vi "Expression Format Example.vi"() -> ()   [LabVIEW 2020, in "Logger Examples.lvlib"]
uses:
  <vilib>/gpm_packages/@cs/event-logger/Examples/Logger Examples.lvlib
  <vilib>/gpm_packages/@cs/event-logger/Source/Composed Log/Types/Log Level.ctl
  <vilib>/gpm_packages/@cs/event-logger/Source/String Formats/String Expression Format/String Expression Format.lvclass/String Expression Format.ctl
  <vilib>/gpm_packages/@cs/event-logger/Source/Composed Log/LoggerReference/LoggerReference.lvclass/LoggerReference.ctl
  601d143e-8928-4a3b-9174-3083e729aaa9.vi
  <vilib>/gpm_packages/@cs/event-logger/Source/String Formats/String Expression Format/Run Formatter.vi
  <vilib>/gpm_packages/@cs/event-logger/Source/Composed Log/LoggerReference/Return Aggregate Queues.vi
  <vilib>/gpm_packages/@cs/event-logger/Source/Composed Log/LoggerReference/Add Aggregate Log.vi
  601d143e-8928-4a3b-9174-3083e729aaa9.vi/f15837f3-2100-4c7f-976a-c76a45bfaa57.vi
  <vilib>/gpm_packages/@cs/event-logger/Source/Composed Log/LoggerReference/Log.vi
  <vilib>/gpm_packages/@cs/event-logger/Source/Composed Log/LoggerReference/Get Valid Event Time.vi
  <vilib>/dlg_ctls.llb/Space Constant.vi
  <vilib>/gpm_packages/@cs/event-logger/Source/Composed Log/LoggerReference/Send Add Sink.vi
  <vilib>/gpm_packages/@cs/event-logger/Source/Composed Log/LoggerReference/Remove Stale Logs.vi
  <vilib>/gpm_packages/@cs/event-logger/Source/String Formats/String Expression Format/String Expression Format.lvclass
  C:/Program Files/National Instruments/LabVIEW 2020/vi.lib/gpm_packages/@cs/event-logger/Source/IStringFormat/IStringFormat.lvclass
  <vilib>/gpm_packages/@cs/event-logger/Source/Text File Sink/Text File Sink.lvclass
  C:/Program Files/National Instruments/LabVIEW 2020/vi.lib/gpm_packages/@cs/event-logger/Source/String Log Sink/String Log Sink.lvclass
  <vilib>/gpm_packages/@cs/event-logger/Source/String Control Sink/String Control Sink.lvclass
  <vilib>/gpm_packages/@cs/event-logger/Source/String Log Sink/String Log Sink.lvclass
  C:/Program Files/National Instruments/LabVIEW 2020/vi.lib/gpm_packages/@cs/event-logger/Source/Composed Log/Log Sink/Log Sink.lvclass
  <vilib>/gpm_packages/@cs/event-logger/Source/Composed Log/Application Logger/Launch Worker Loop.vi
  <vilib>/gpm_packages/@cs/event-logger/Source/Composed Log/LoggerReference/Initialize Logger Instance.vi
  <vilib>/gpm_packages/@cs/event-logger/Source/Composed Log/LoggerReference/LoggerReference.lvclass
  <vilib>/gpm_packages/@cs/event-logger/Source/Composed Log/IErrorFormat/IErrorFormat.lvclass
  <vilib>/gpm_packages/@cs/event-logger/Source/Composed Log/Log Sink/Log Sink.lvclass
  <vilib>/gpm_packages/@cs/event-logger/Source/Composed Log/Composed Log.lvlib
  <vilib>/gpm_packages/@cs/event-logger/Source/Composed Log/ILogFilter/ILogFilter.lvclass
panel:
  in  "Log Error":bool
  in  "Error Information":string
  in  "Error Code":i32
  in  "Event Level":T1(ring)
  out "Event - %s[EVT]  - Occured at <%T>[TIME] From %s[ID], Level %s[LVL]":string
  out "%<%A at %H:%M:%S>T[TIME] -- %s[EVT]":string
  out "<%T>[TIME]<%s[LVL]-%s[ID]><%s>[EVT]":string
  in  "Data To Log":string
  in  "Source":string="User"
  in  "Log":bool
  # "Run the VI. Note the different formats - each string indicator is displaying the same event with different string format."
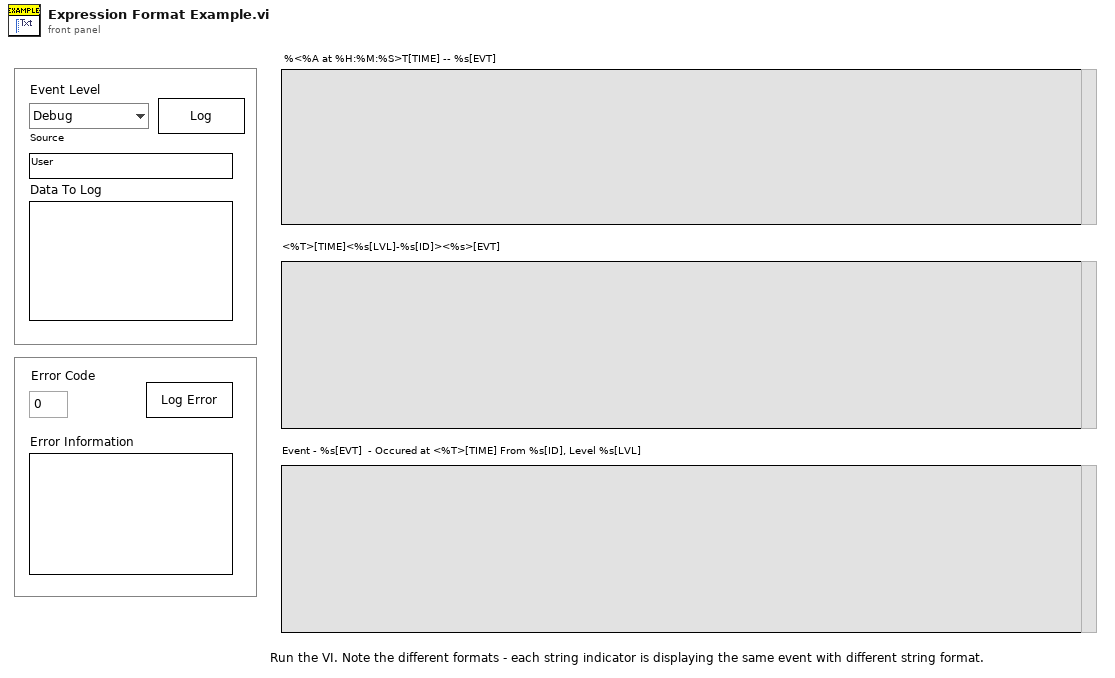
[diagram p1: front panel]
types:
  T1 = enum16{"Debug", "Info", "Warning", "Error", "Critical"}
  T2 = typedef "Composed Log.lvlib/Log Level.ctl" = enum16{"Debug", "Info", "Warning", "Error", "Critical"}
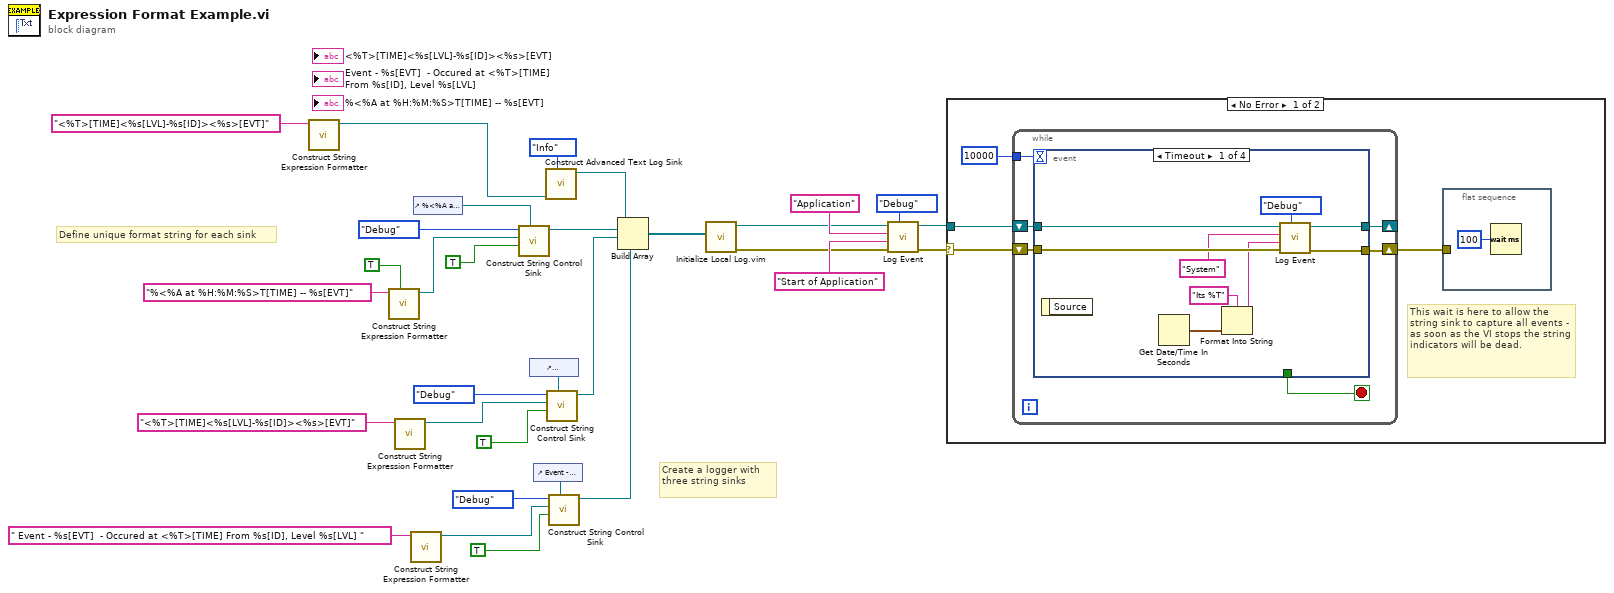
[diagram p0: block diagram]
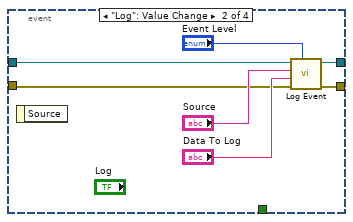
[diagram p2: hidden frame]
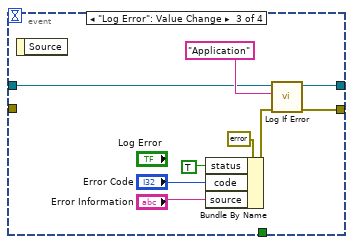
[diagram p3: hidden frame]
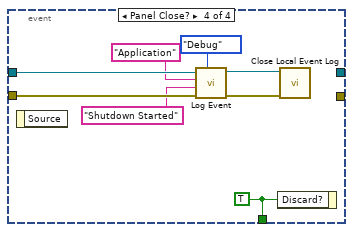
[diagram p4: hidden frame]
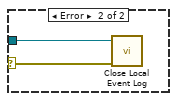
[diagram p5: hidden frame]
diagram:
  # "Define unique format string for each sink"
  # "Create a logger with three string sinks"
  n1 = call <vilib>:"Construct String Expression Formatter.vi"("Format Specifier"="<%T>[TIME]<%s[LVL]-%s[ID]><%s>[EVT]") -> ("String Expression Format out"=w1:refnum<class "String Expression Format.lvclass">)  [unwired: 9 in, 1 out]
  n2 = call <vilib>:"Construct String Expression Formatter.vi"("Append EOL?"=TRUE, "Format Specifier"="%<%A at %H:%M:%S>T[TIME] -- %s[EVT]") -> ("String Expression Format out"=w14:refnum<class "String Expression Format.lvclass">)  [unwired: 8 in, 1 out]
  n3 = call <vilib>:"Construct String Expression Formatter.vi"("Format Specifier"="<%T>[TIME]<%s[LVL]-%s[ID]><%s>[EVT]") -> ("String Expression Format out"=w11:refnum<class "String Expression Format.lvclass">)  [unwired: 9 in, 1 out]
  n4 = call <vilib>:"Construct String Expression Formatter.vi"("Format Specifier"=" Event - %s[EVT]  - Occured at <%T>[TIME] From %s[ID], Level %s[LVL] ") -> ("String Expression Format out"=w7:refnum<class "String Expression Format.lvclass">)  [unwired: 9 in, 1 out]
  n5 = control-ref of="%<%A at %H:%M:%S>T[TIME] -- %s[EVT]"() -> (w27:refnum<vi>)
  n6 = call <vilib>:"Construct String Control Sink.vi"("Str Refnum"=w27, "AutoScroll?(F)"=TRUE, "LogFormat"=w14, "LogLevel"=Log_Level."Debug") -> ("String Control Sink out"=w22:refnum<class "String Control Sink.lvclass">)  [unwired: 7 in]
  n7 = control-ref of="<%T>[TIME]<%s[LVL]-%s[ID]><%s>[EVT]"() -> (w29:refnum<vi>)
  n8 = control-ref of="Event - %s[EVT]  - Occured at <%T>[TIME] From %s[ID], Level %s[LVL]"() -> (w23:refnum<vi>)
  n9 = call <vilib>:"Construct Advanced Text Log Sink.vi"("LogLevel"=Log_Level."Info", "StringFormat"=w1) -> ("Text File Sink out"=w4:refnum<class "Text File Sink.lvclass">)  [unwired: 9 in]
  n10 = call <vilib>:"Construct String Control Sink.vi"("Str Refnum"=w29, "AutoScroll?(F)"=TRUE, "LogFormat"=w11, "LogLevel"=Log_Level."Debug") -> ("String Control Sink out"=w10:refnum<class "String Control Sink.lvclass">)  [unwired: 7 in]
  n11 = call <vilib>:"Construct String Control Sink.vi"("Str Refnum"=w23, "AutoScroll?(F)"=TRUE, "LogFormat"=w7, "LogLevel"=Log_Level."Debug") -> ("String Control Sink out"=w6:refnum<class "String Control Sink.lvclass">)  [unwired: 7 in]
  n12 = Build Array(w4, w22, w10, w6) -> (w5:refnum<class "String Log Sink.lvclass">[])
  n13 = call "Initialize Local Log.vim"("Startup Sink(s)"=w5) -> ("error out"=w18:errorcluster, "Log Instance Reference"=w17:refnum<class "LoggerReference.lvclass">)  [unwired: 8 in, 1 out]
  n14 = call <vilib>:"Log Event.vi"("Event Level"=Log_Level."Debug", "error in (no error)"=w18, "Data To Log"="Start of Application", "SourceID"="Application", "Log Instance"=w17) -> ("error out"=w16:errorcluster, "Log Instance Out"=w15:refnum<class "LoggerReference.lvclass">)  [unwired: 5 in]
  n15 = case shown="No Error" w16 {
    selector: w16 -> [w34 w76]
    tunnel: w15 -> [w35 w77]
    frame No Error {
      # "This wait is here to allow the string sink to capture all events - as soon as the VI stops the string indicators will be dead."
      n16 = while {
        shift-right: [w40] -> _
        shift-left: w35 -> [w41]
        shift-right: [w38] -> w32
        shift-left: w34 -> [w39]
        tunnel: 10000 -> [w37]
        stop <- w42 stop-if-true
        n17 = event shown="[0] Timeout" {
          selector: _ -> [_ _ _ _]
          dyn-events: _ -> [_ _ _ _]
          timeout: w37 -> [_ _ _ _]
          tunnel: [_ _ _ w75] -> w42
          tunnel: w41 -> [w51 w55 w61 w73]
          tunnel: [w50 w53 w59 _] -> w40
          tunnel: w39 -> [w48 w52 _ w74]
          tunnel: [w47 w54 w60 _] -> w38
          event Timeout {
            n18 = event-data() -> ()  [unwired: 1 in, 1 out]
            n19 = Get Date/Time In Seconds() -> (seconds since 1Jan1904=w45:timestamp)
            n20 = Format Into String(format string="Its %T" ("Log Message"), w45) -> (resulting string=w43:string)  [unwired: 2 in, 1 out]
            n21 = call <vilib>:"Log Event.vi"("Event Level"=Log_Level."Debug", "error in (no error)"=w48, "Data To Log"=w43, "SourceID"="System" ("Event Source"), "Log Instance"=w51) -> ("error out"=w47:errorcluster, "Log Instance Out"=w50:refnum<class "LoggerReference.lvclass">)  [unwired: 5 in]
          }
          event "Log": Value Change {
            n22 = event-data() -> ()  [unwired: 1 in, 1 out]
            n23 = call <vilib>:"Log Event.vi"("Event Level"="Event Level", "error in (no error)"=w52, "Data To Log"="Data To Log", "SourceID"="Source", "Log Instance"=w55) -> ("error out"=w54:errorcluster, "Log Instance Out"=w53:refnum<class "LoggerReference.lvclass">)  [unwired: 5 in]
          }
          event "Log Error": Value Change {
            n24 = event-data() -> ()  [unwired: 1 in, 1 out]
            n25 = Bundle By Name(cluster=errorcluster {"status"=FALSE, "code"=0, "source"=""} ("Error In"), "status"=TRUE, "code"="Error Code", "source"="Error Information") -> (w65:errorcluster)
            n26 = call <vilib>:"Log If Error.vi"("Error In"=w65, "SourceID"="Application" ("Source"), "Log Instance"=w61) -> ("error out"=w60:errorcluster, "Log Instance Out"=w59:refnum<class "LoggerReference.lvclass">)  [unwired: 7 in]
          }
          event Panel Close? {
            w75 = TRUE ("Discard?")
            n27 = event-data() -> ()  [unwired: 1 in, 1 out]
            n28 = call <vilib>:"Log Event.vi"("Event Level"=Log_Level."Debug", "error in (no error)"=w74, "Data To Log"="Shutdown Started", "SourceID"="Application", "Log Instance"=w73) -> ("error out"=w72:errorcluster, "Log Instance Out"=w71:refnum<class "LoggerReference.lvclass">)  [unwired: 5 in]
            n29 = event-data("Discard?"=w75) -> ()  [unwired: 1 in, 1 out]
            n30 = call <vilib>:"Close Local Event Log.vi"("error in (no error)"=w72, "Log Instance"=w71) -> ()  [unwired: 9 in, 1 out]
          }
        }
      }
      n31 = flat-sequence {
        tunnel: w32 -> [_]
        frame #0 {
          n32 = Wait (ms)(milliseconds to wait=u32 100) -> ()  [unwired: 1 out]
        }
      }
    }
    frame Error {
      n33 = call <vilib>:"Close Local Event Log.vi"("error in (no error)"=w76, "Log Instance"=w77) -> ()  [unwired: 9 in, 1 out]
    }
  }
